vi "SLSC Scripting Constants.vi"() -> ()   [LabVIEW 2017, in "SLSC Switch Scripting.lvlib"]
doc: "Use this Global VI to access the GUIDs assigned to the page resources of the Custom Device."
uses:
  SLSC Switch Scripting.lvlib
panel:
  in  "Tab Control":T1(tab)=enum."Properties"
  in  "SLSC Sw:Status Section":string="Status"
  in  "SLSC Sw:Endpoint Section":string="Endpoint Configuration"
  in  "SLSC Sw:Prop:Model":string="Model"
  in  "SLSC Sw:Prop:Resource":string="Resource"
  in  "SLSC Sw:Prop:Topology":string="Topology"
  in  "SLSC Sw:Prop:Capabilities":string="Capabilities"
  in  "Compiled.Settings":string="Compiled.Settings"
  in  "GUID.Status":string="80DE2635-1DC5-B67A-CA46-E31C1EC1F9C0"
  in  "ChanList.HeartbeatChan":string="Heartbeat"
  in  "ChanList.StatusCode":string="Status code"
  in  "Desc.HeartbeatChan":string="Running count used for debugging. If this channel continues to increment, the custom device is still executing."
  in  "Desc.StatusCode":string="Status code of the custom device. A negative value indicates failure. A positive value indicates warning."
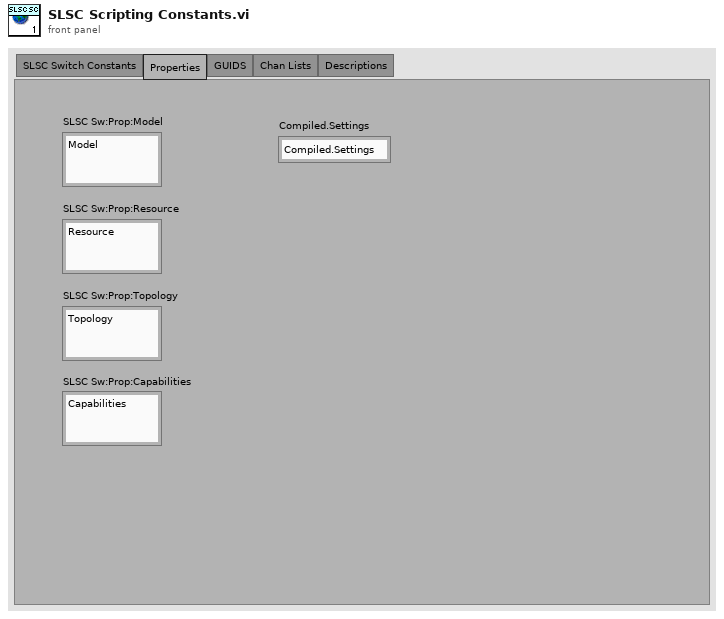
[diagram p1: front panel]
types:
  T1 = enum32{"SLSC Switch Constants", "Properties", "GUIDS", "Chan Lists", "Descriptions"}
diagram:
